vi "Calculate laser rates.vi"(7 "Tasks":T1={"CLk"="CRDS Red Clk", "AI"="CRDS Red AI", "DO"="CRD Red Laser Output"}, 8 "error in (no error)":errorcluster, 9 "Laser DC (%)":dbl, 10 "Laser Rep (Hz)":dbl, 11 "DAQ":T2={"Rate (MHz)"=4.0, "Laser Rep (Hz)"=2000.0, "Laser DC (%)"=0.5}) -> (0 "error out":errorcluster, 1 "Laser DC":dbl, 2 "Laser Rep (Hz)":dbl, 3 "DAQ":T2, 5 "Tasks out":T1={"CLk"="CRDS Red Clk", "AI"="CRDS Red AI", "DO"="CRD Red Laser Output"})   [LabVIEW 2014, in "eCRDS Library.lvlib" / "Update Laser rate and DC.lvclass"]
uses:
  Update Laser rate and DC.lvclass
  <vilib>/DAQmx/configure/timing.llb/DAQmx Timing (Implicit).vi
  <resource>/objmgr/daqmx.rc
panel:
  out "error out 2":errorcluster
  out "Low":dbl
  out "High":dbl
  out "Samples":i32
  out "CO.Pulse.LowTime":dbl
  out "CO.Pulse.HighTime":dbl
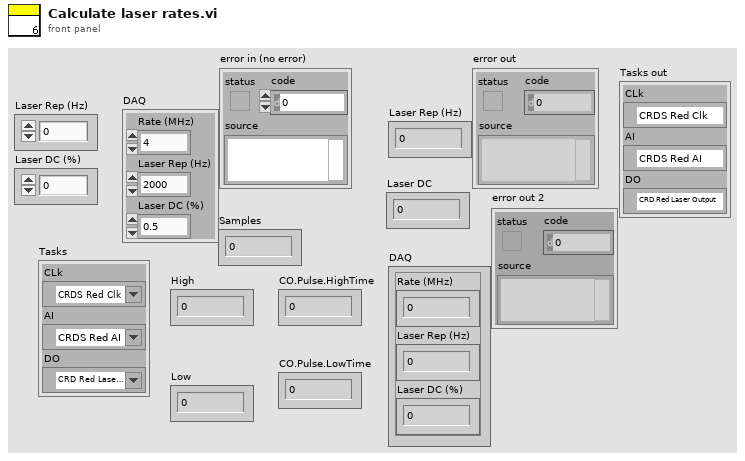
[diagram p1: front panel]
types:
  T1 = cluster{"CLk":refnum<k21>, "AI":refnum<k21>, "DO":refnum<k21>}
  T2 = cluster{"Rate (MHz)":dbl, "Laser Rep (Hz)":dbl, "Laser DC (%)":dbl}
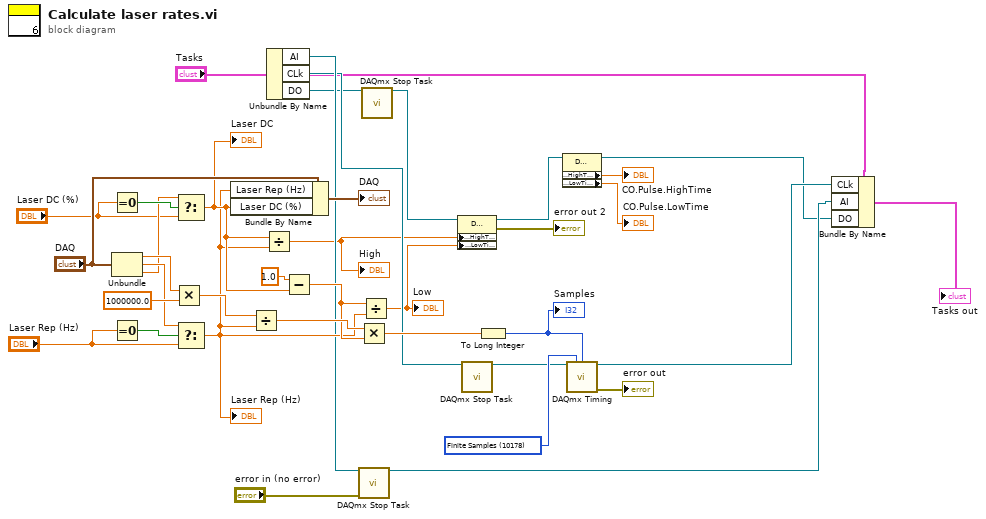
[diagram p0: block diagram]
diagram:
  w18 = 10178 items=["Finite Samples"=10178, "Continuous Samples"=10123, "Hardware Timed Single Point"=12522] ("sample mode")
  n1 = Equal To 0?(x="Laser DC (%)") -> (x = 0?=w30:bool)
  n2 = Unbundle("DAQ") -> ("Rate (MHz)"=w27:dbl, "Laser Rep (Hz)"=w32:dbl, "Laser DC (%)"=w21:dbl)
  n3 = Equal To 0?(x="Laser Rep (Hz)") -> (x = 0?=w33:bool)
  n4 = Multiply(x=w27, y=1000000.0) -> (x*y=w23:dbl)
  n5 = Select(t=w21, s=w30, f="Laser DC (%)") -> (s? t:f=w24:dbl)
  "Laser DC" <- w24
  n6 = Select(t=w32, s=w33, f="Laser Rep (Hz)") -> (s? t:f=w22:dbl)
  "Laser Rep (Hz)" <- w22
  n7 = Bundle By Name(cluster="DAQ", "Laser Rep (Hz)"=w22, "Laser DC (%)"=w24) -> (→"DAQ":T2)
  n8 = Divide(x=w23, y=w22) -> (x/y=w35:dbl)
  n9 = Divide(x=w24, y=w22) -> (x/y=w6:dbl)
  "High" <- w6
  n10 = Unbundle By Name("Tasks") -> ("AI"=w19:refnum<k21>, "CLk"=w11:refnum<k21>, "DO"=w10:refnum<k21>)
  n11 = Subtract(x=1.0, y=w24) -> (x-y=w25:dbl)
  n12 = Multiply(x=w35, y=w25) -> (x*y=w34:dbl)
  n13 = call <vilib>:"DAQmx Stop Task.vi"("task/channels in"=w19, "error in"="error in (no error)") -> ("task out"=w2:refnum<k21>)  [unwired: 12 in, 1 out]
  n14 = Divide(x=w25, y=w22) -> (x/y=w7:dbl)
  "Low" <- w7
  n15 = call <vilib>:"DAQmx Stop Task.vi"("task/channels in"=w10) -> ("task out"=w9:refnum<k21>)  [unwired: 13 in, 1 out]
  n16 = property class="DAQmx Channel"(reference=w9, "CO.Pulse.HighTime"=w6, "CO.Pulse.LowTime"=w7) -> (reference out=w13:refnum<k21>, error out=→"error out 2":errorcluster)  [unwired: 1 in]
  n17 = call <vilib>:"DAQmx Stop Task.vi"("task/channels in"=w11) -> ("task out"=w8:refnum<k21>)  [unwired: 13 in, 1 out]
  n18 = To Long Integer(number=w34) -> (32bit integer=w26:i32)
  "Samples" <- w26
  n19 = property class="DAQmx Channel"(reference=w13) -> (reference out=w1:refnum<k21>, "CO.Pulse.HighTime"=→"CO.Pulse.HighTime":dbl, "CO.Pulse.LowTime"=→"CO.Pulse.LowTime":dbl)  [unwired: 1 in, 1 out]
  n20 = call-poly <vilib>:"DAQmx Timing.vi"("task/channels in"=w8, "sample mode"=w18, "samples per channel"=w26) -> ("task out"=w3:refnum<k21>, "error out"=→"error out":errorcluster)  [unwired: 11 in]
  n21 = Bundle By Name(cluster="Tasks", "CLk"=w3, "AI"=w2, "DO"=w1) -> (→"Tasks out":T1)
